vi "Write RLNA URL.vi"(8 "error in (no error)":errorcluster, 10 "RLNA URL":string, 11 "Test LNA in":refnum<class "TestLNA.lvclass">) -> (0 "error out":errorcluster, 3 "Test LNA out":refnum<class "TestLNA.lvclass">)   [LabVIEW 2014, in "TestLNA.lvlib" / "TestLNA.lvclass"]
uses:
  TestLNA.lvclass
  TestLNA.lvclass/TestLNA.ctl
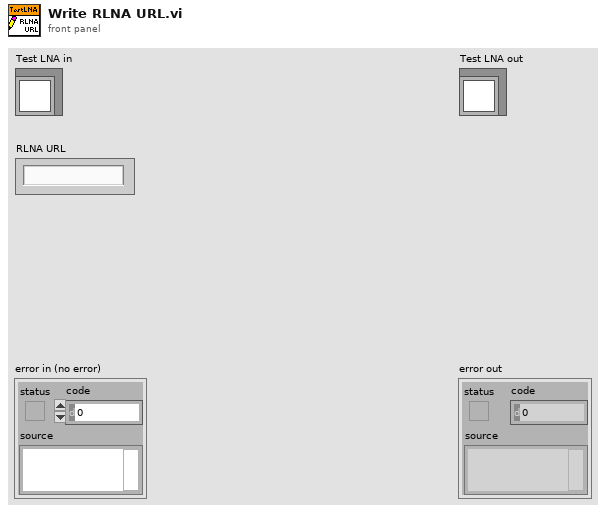
[diagram p1: front panel]
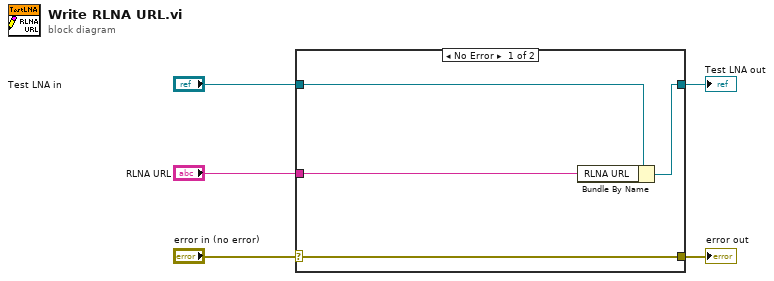
[diagram p0: block diagram]
diagram:
  n1 = case shown="No Error" "error in (no error)" {
    selector: "error in (no error)" -> [w9 w10]
    tunnel: [w9 w10] -> w4
    tunnel: [w7 w11] -> w2
    tunnel: "Test LNA in" -> [w8 w11]
    tunnel: "RLNA URL" -> [w6 _]
    frame No Error {
      n2 = Bundle By Name(cluster=w8, "RLNA URL"=w6) -> (w7:refnum<class "TestLNA.lvclass">)
    }
    frame Error {
    }
  }
  "error out" <- w4
  "Test LNA out" <- w2
